vi "Read message.vi"(8 "error in (no error)":errorcluster, 11 "message_text in":refnum<class "message_text.lvclass">) -> (0 "error out":errorcluster, 2 "message":T1, 3 "message_text out":refnum<class "message_text.lvclass">)   [LabVIEW 2020, in "message_text.lvclass"]
uses:
  message_text.lvclass
  message.ctl
  message_text.lvclass/message_text.ctl
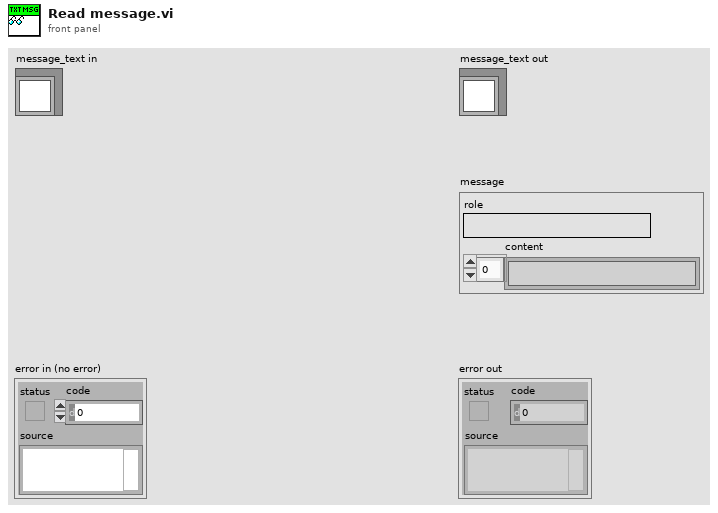
[diagram p1: front panel]
types:
  T1 = typedef "message_text.lvclass/message.ctl" = cluster{"role":string, "content":string[]}
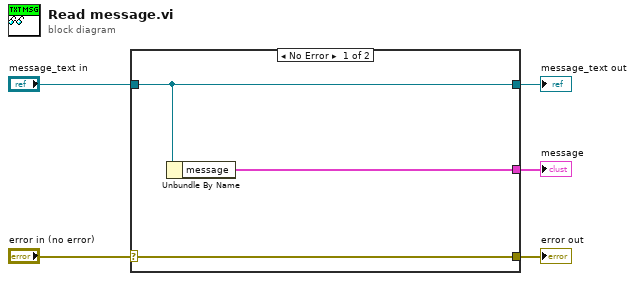
[diagram p0: block diagram]
diagram:
  n1 = case shown="No Error" "error in (no error)" {
    selector: "error in (no error)" -> [w8 w9]
    tunnel: [w8 w9] -> w4
    tunnel: [w7 w10] -> w2
    tunnel: "message_text in" -> [w7 w10]
    tunnel: [w6 _] -> w1
    frame No Error {
      n2 = Unbundle By Name(w7) -> ("message"=w6:T1)
    }
    frame Error {
    }
  }
  "error out" <- w4
  "message_text out" <- w2
  "message" <- w1
